vi "rqp_Start Polling.vi"(4 "Show in Debugger?":bool=TRUE, 6 "Message Priority":T1=enum."Normal", 7 "Caller in":refnum<class "Worker.lvclass">, 8 "error in":errorcluster, 10 "Data in":T2, 11 "Base Hardware in":refnum<class "Base Hardware.lvclass">) -> (0 "error out":errorcluster, 3 "dup Base Hardware out":refnum<class "Base Hardware.lvclass">)   [LabVIEW 2020, in "Abstract Hardware.lvlib" / "Base Hardware.lvclass"]
doc: "This VI sends a <b>Public API Request</b> message to an MHL case of the Worker that owns this VI.\n---\nWorkers Public API Request Case"
uses:
  Base Hardware.lvclass
  C:/Program Files (x86)/National Instruments/LabVIEW 2020/vi.lib/addons/_Workers/Library/Classes/Worker/Worker.lvclass
  <vilib>/addons/_Workers/Library/Classes/Worker/Worker.lvclass
  rqp_Start Polling.ctl
  <vilib>/addons/_Workers/Library/Classes/Message/Priority.ctl
  <vilib>/addons/_Workers/Library/Case Label.ctl
  <vilib>/addons/_Workers/Library/Classes/Message/Message.lvclass
  <vilib>/addons/_Workers/Library/Classes/Worker/Worker.lvclass/Worker.ctl
  <vilib>/addons/_Workers/Library/Classes/Message/Message.lvclass/Message.ctl
  <vilib>/addons/_Workers/Library/Classes/Message/Write Time Stamp.vi
  <vilib>/addons/_Workers/Library/Classes/Message/Write Sender WID.vi
  <vilib>/addons/_Workers/Library/Classes/Message/Write Data.vi
  <vilib>/addons/_Workers/Library/Classes/Message/Write Recipient Case.vi
  <vilib>/addons/_Workers/Library/Classes/Message/Message Time Stamp.vi
  <vilib>/addons/_Workers/Library/Classes/Message/Write Sender Case.vi
  <vilib>/addons/_Workers/Library/Classes/Worker/Read Message.vi
  <vilib>/addons/_Workers/Library/Classes/Message/Read Recipient Case.vi
  <vilib>/addons/_Workers/Library/Classes/Message/Write Auxiliary.vi
  <vilib>/addons/_Workers/Library/Classes/Worker/Read WID.vi
  <vilib>/Utility/High Resolution Relative Seconds.vi
  <vilib>/addons/_Workers/Library/Classes/Message Queue/Message Queue.lvclass
  <vilib>/addons/_Workers/Library/Workers.lvlib
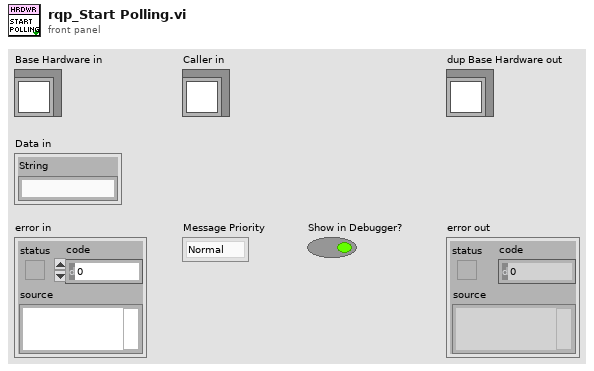
[diagram p1: front panel]
types:
  T1 = typedef "Workers.lvlib/Message.lvclass/Priority.ctl" = enum16{"Low", "Normal", "High"}
  T2 = typedef "Abstract Hardware.lvlib/Base Hardware.lvclass/rqp_Start Polling.ctl" = cluster{"String":string}
  T3 = typedef "Workers.lvlib/Case Label.ctl" = string
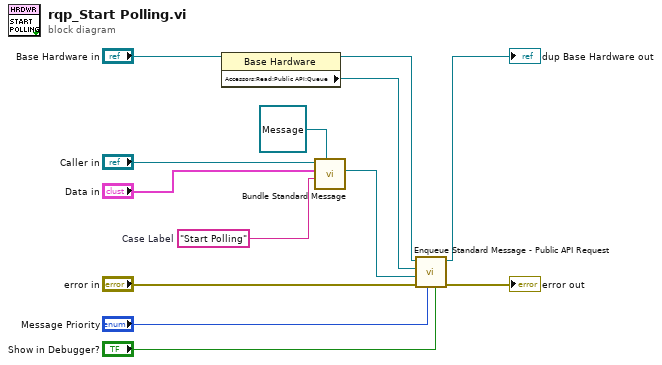
[diagram p0: block diagram]
diagram:
  w1 = T3 "Start Polling"  # Case Label
  n1 = property class="Base Hardware"(reference="Base Hardware in") -> (reference out=w9:refnum<class "Base Hardware.lvclass">, "Accessors:Read:Public API:Queue"=w2:refnum<class "Message Queue.lvclass">)  [unwired: 1 in, 1 out]
  n2 = call <vilib>:"Bundle Standard Message.vi"("Message"=refnum<class "Message.lvclass"> refnum, "Case"=w1, "Data"="Data in", "Worker"="Caller in") -> ("Message out"=w5:refnum<class "Message.lvclass">)  [unwired: 6 in, 1 out]
  n3 = call <vilib>:"Enqueue Standard Message - Public API Request.vi"("Send Message to Debugger? (T)"="Show in Debugger?", "Priority (Normal)"="Message Priority", "error in (no error)"="error in", "Message"=w5, "Message Queue"=w2, "Worker in"=w9) -> ("error out"=→"error out":errorcluster, "dup Worker out"=→"dup Base Hardware out":refnum<class "Base Hardware.lvclass">)  [unwired: 4 in]
